vi "Get MathFunction Name.vi"(8 "error in (no error)":errorcluster, 11 "Add in":refnum<class "Add.lvclass">) -> (0 "error out":errorcluster, 2 "MathFunction Name":string, 3 "Add out":refnum<class "Add.lvclass">)   [LabVIEW 2019, in "lv-classprovidershell-example.lvlib" / "Add.lvclass"]
uses:
  Add.lvclass
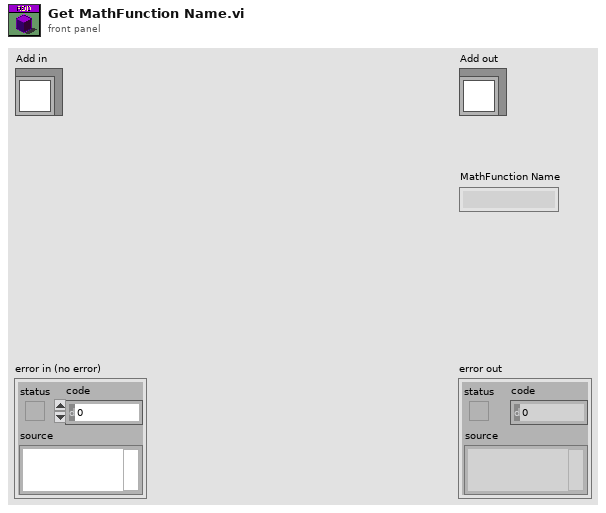
[diagram p1: front panel]
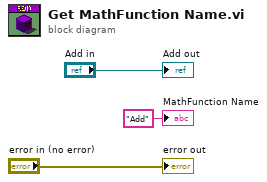
[diagram p0: block diagram]
diagram:
  "error out" <- "error in (no error)"
  "Add out" <- "Add in"
  "MathFunction Name" <- "Add" ("MathFunction Name")
